vi "save.vi"(8 "error in (no error)":errorcluster, 10 "Path":path, 11 "VGS_Project in":refnum<class "VGS_Project.lvclass">) -> (0 "error out":errorcluster, 1 "Time, ms":u32, 3 "VGS_Project out":refnum<class "VGS_Project.lvclass">)   [LabVIEW 2022 SP3, in "LV_VGS.lvlib" / "VGS_Project.lvclass"]
uses:
  VGS_Project.lvclass
  VGS_Project.lvclass/VGS_Project.ctl
  C:/Users/Andrey/Desktop/hajo/LV_VGS/vgs_project.dll
  vgs_project.dll
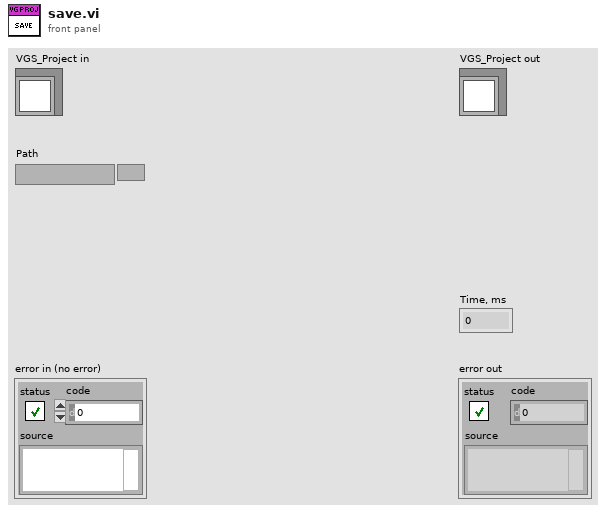
[diagram p1: front panel]
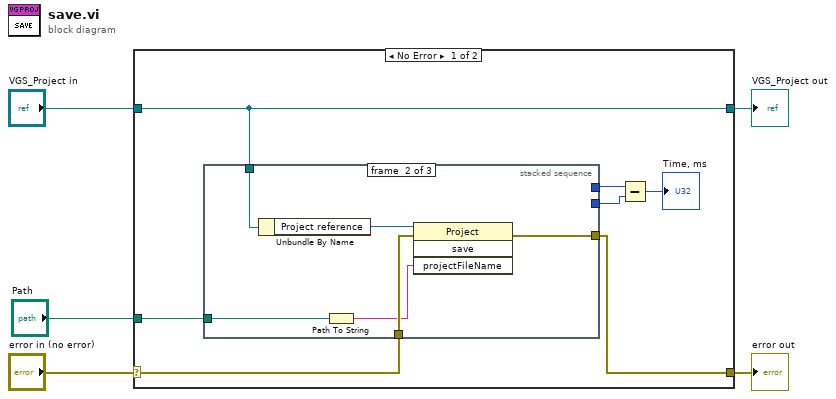
[diagram p0: block diagram]
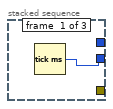
[diagram p2: hidden frame]
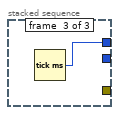
[diagram p3: hidden frame]
diagram:
  n1 = case shown="No Error" "error in (no error)" {
    selector: "error in (no error)" -> [w11 w22]
    tunnel: [w10 w22] -> w4
    tunnel: [w12 w21] -> w2
    tunnel: "VGS_Project in" -> [w12 w21]
    tunnel: "Path" -> [w9 _]
    frame No Error {
      n2 = stacked-sequence {
        tunnel: w12 -> [_ w19 _]
        tunnel: w11 -> [_ w17 _]
        tunnel: [_ w16 _] -> w10
        tunnel: w9 -> [_ w15 _]
        tunnel: [w13 _ _] -> w7
        tunnel: [_ _ w20] -> w8
        frame #0 {
          n3 = Tick Count (ms)() -> (millisecond timer value=w13:u32)
        }
        frame #1 {
          n4 = Unbundle By Name(w19) -> ("Project reference"=w18:refnum<k24>)
          n5 = Path To String(path=w15) -> (string=w14:string)
          n6 = invoke class="Project" method="save"(reference=w18, error in=w17, "projectFileName"=w14) -> (error out=w16:errorcluster)  [unwired: 1 in, 3 out]
        }
        frame #2 {
          n7 = Tick Count (ms)() -> (millisecond timer value=w20:u32)
        }
      }
      n8 = Subtract(x=w8, y=w7) -> (x-y=→"Time, ms":u32)
    }
    frame Error {
    }
  }
  "error out" <- w4
  "VGS_Project out" <- w2
